vi "Create Framework.vi"(8 "error in (no error)":errorcluster, 11 "Application Data in":T1) -> (0 "error out":errorcluster, 2 "new item tag":string, 3 "Application Data Out":T1)   [LabVIEW 2017, in "DSF Core.lvlib"]
uses:
  DSF Core.lvlib
  Main VI/Application Data.ctl
  LabVIEW-Memory/Source/Classes/Pointer/Pointer.lvclass
  Classes/Framework/Framework.lvclass
  Buffer Reader/Buffer Data.ctl
  Classes/Buffer/Buffer.lvclass
  Classes/Transfer Group Status/Status.lvclass
  Typedefs/DSF Data Type.ctl
  Typedefs/DSF Engine Channel Configuration.ctl
  Typedefs/DSF Settings Info.ctl
  Typedefs/DSF Byte Order.ctl
  Typedefs/DSF Engine Framework Configuration.ctl
  Typedefs/DSF Engine Plugin Configuration.ctl
  Typedefs/DSF Timing Info.ctl
  Typedefs/DSF Engine Plugin Thread Configuration.ctl
  Typedefs/DSF Engine Transfer Group Configuration.ctl
  Typedefs/DSF Direction.ctl
  Typedefs/DSF Engine Transfer Configuration.ctl
  Typedefs/DSF Timeout Behavior.ctl
  Classes/Framework/Framework.lvclass/Framework.ctl
  Classes/Framework Status/Framework Status.lvclass/Framework Status.ctl
  ID to Tree Items/Tree Item Type.ctl
  Classes/Framework Status/Framework Status.lvclass
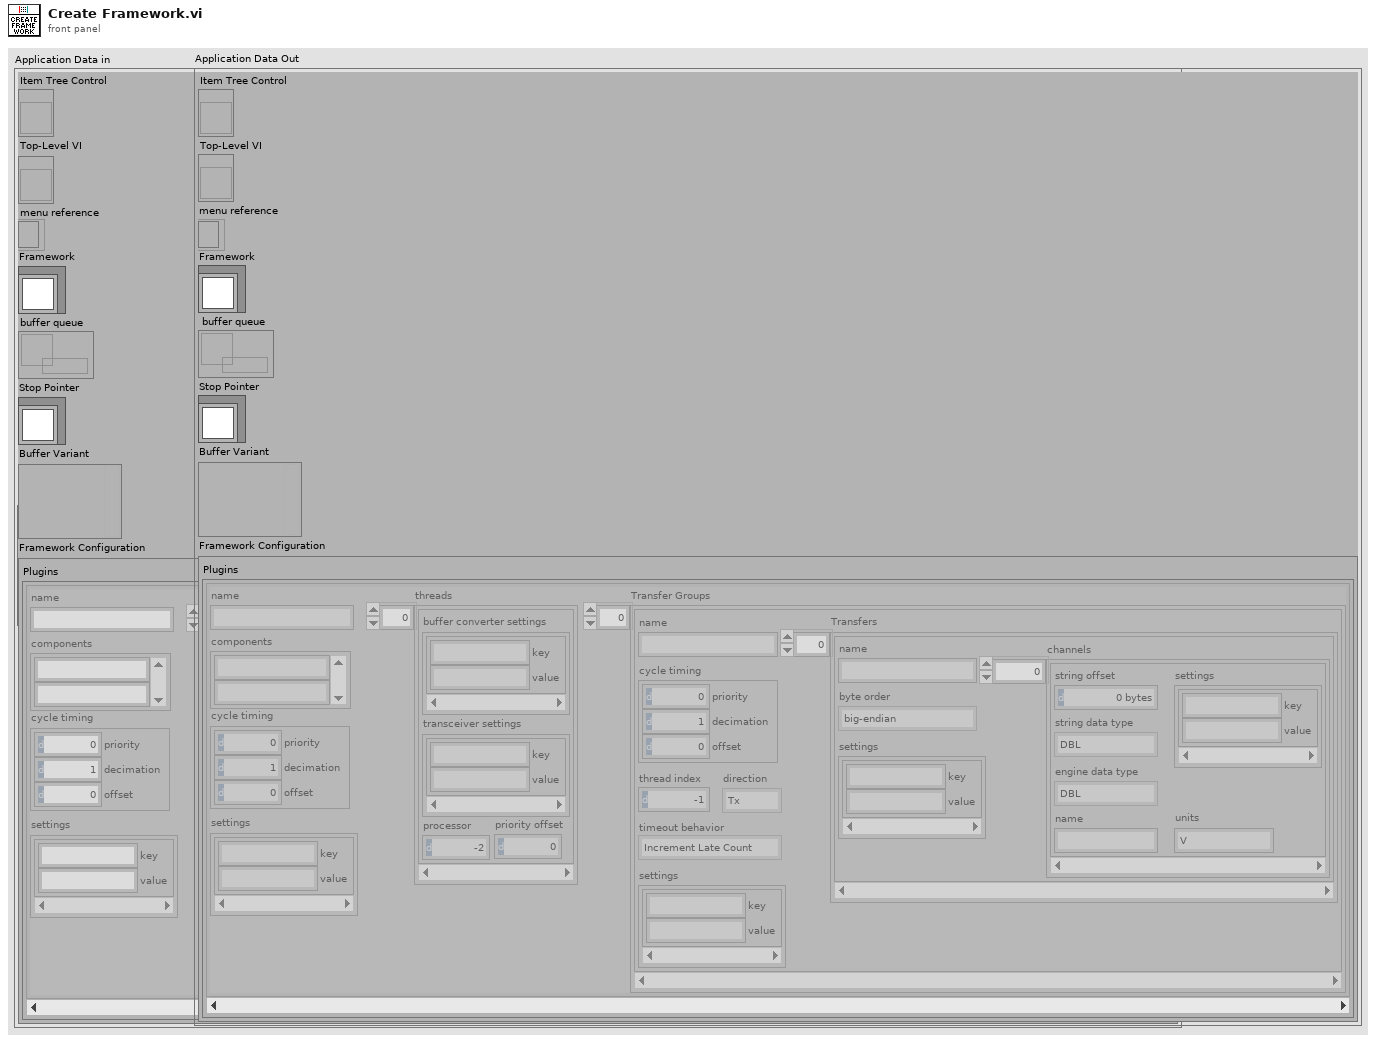
[diagram p1: front panel]
types:
  T1 = typedef "DSF Core.lvlib/Application Data.ctl" = cluster{"Item Tree Control":refnum<vi>, "Top-Level VI":refnum<vi>, "menu reference":refnum<k9>, "Framework":refnum<class "Framework.lvclass">, "buffer queue":refnum<queue>, "Stop Pointer":refnum<class "Pointer.lvclass">, "Buffer Variant":variant, "Framework Configuration":T2}
  T2 = typedef "DSF Core.lvlib/DSF Engine Framework Configuration.ctl" = cluster{"Plugins":T3[]}
  T3 = typedef "DSF Core.lvlib/DSF Engine Plugin Configuration.ctl" = cluster{"name":string, "components":string[], "cycle timing":T4, "threads":T5[], "Transfer Groups":T7[], "settings":T6}
  T4 = typedef "DSF Core.lvlib/DSF Timing Info.ctl" = cluster{"priority":u64, "decimation":u64, "offset":u64}
  T5 = typedef "DSF Core.lvlib/DSF Engine Plugin Thread Configuration.ctl" = cluster{"buffer converter settings":T6, "transceiver settings":T6, "processor":i32, "priority offset":i16}
  T6 = typedef "DSF Core.lvlib/DSF Settings Info.ctl" = cluster{"key":string, "value":string}[]
  T7 = typedef "DSF Core.lvlib/DSF Engine Transfer Group Configuration.ctl" = cluster{"name":string, "direction":T8, "cycle timing":T4, "thread index":i32, "settings":T6, "Transfers":T9[], "timeout behavior":T13}
  T8 = typedef "DSF Core.lvlib/DSF Direction.ctl" = enum8{"Tx", "Rx"}
  T9 = typedef "DSF Core.lvlib/DSF Engine Transfer Configuration.ctl" = cluster{"name":string, "byte order":T10, "settings":T6, "channels":T11[]}
  T10 = typedef "DSF Core.lvlib/DSF Byte Order.ctl" = enum8{"big-endian", "little-endian"}
  T11 = typedef "DSF Core.lvlib/DSF Engine Channel Configuration.ctl" = cluster{"string offset":u64, "string data type":T12, "engine data type":T12, "name":string, "settings":T6, "units":string}
  T12 = typedef "DSF Core.lvlib/DSF Data Type.ctl" = enum8{"Bool", "SGL", "DBL", "I8", "I16", "I32", "I64", "U8", "U16", "U32", "U64"}
  T13 = typedef "DSF Core.lvlib/DSF Timeout Behavior.ctl" = enum8{"Increment Late Count", "Throw Error"}
  T14 = typedef "DSF Core.lvlib/Buffer Data.ctl" = cluster{"Buffer":refnum<class "Buffer.lvclass">, "Status":refnum<class "Status.lvclass">, "decimation":u64, "avg bandwidth":dbl, "data type":T12, "units":string, "channels":T11[], "channel":bool, "engine (T) / string (F)":bool, "byte order":T10}
  T15 = typedef "DSF Core.lvlib/Tree Item Type.ctl" = enum16{"Framework", "Plugin Group", "Plugin", "Group", "Transfer", "Buffer", "Channel"}
  T16 = typedef "DSF Core.lvlib/Tree Item.ctl" = cluster{"Left Cell String":string, "Child Text":string[], "Child Tag":string, "Glyph Index":i32}
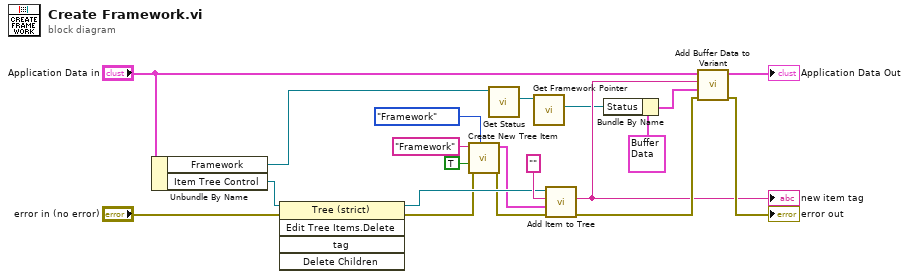
[diagram p0: block diagram]
diagram:
  n1 = Unbundle By Name("Application Data in") -> ("Framework"=w4:refnum<class "Framework.lvclass">, "Item Tree Control"=w12:refnum<vi>)
  n2 = invoke class="Tree (strict)" method="Edit Tree Items.Delete"(reference=w12, error in="error in (no error)") -> (reference out=w19:refnum<vi>, error out=w18:errorcluster)  [unwired: 3 in, 3 out]
  n3 = call "Create New Tree Item.vi"("Item Type"=Tree_Item_Type."Framework", "error in"=w18, "found?"=TRUE, "Left Cell String"="Framework") -> ("error out"=w17:errorcluster, "Item"=w16:T16)  [unwired: 6 in]
  n4 = call "Get Status.vi"("Framework in"=w4) -> ("Status"=w3:refnum<class "Framework Status.lvclass">)  [unwired: 9 in, 1 out]
  n5 = call "Get Framework Pointer.vi"("Framework Status in"=w3) -> ("framework pointer"=w2:refnum<class "Status.lvclass">)  [unwired: 9 in, 1 out]
  n6 = call "Add Item to Tree.vi"("error in (no error)"=w17, "Item"=w16, "parent tag"="", "TreeControl in"=w19) -> ("error out"=w7:errorcluster, "new item tag"=w6:string)  [unwired: 5 in, 1 out]
  "new item tag" <- w6
  n7 = Bundle By Name(cluster=T14 {"Buffer"=refnum, "Status"=refnum, "decimation"=0, "avg bandwidth"=0.0, "data type"=enum."Bool", "units"="", "channels"=[], "channel"=FALSE, "engine (T) / string (F)"=FALSE, "byte order"=enum."little-endian"} ("Buffer data"), "Status"=w2) -> (w1:T14)
  n8 = call "Add Buffer Data to Variant.vi"("error in (no error)"=w7, "Buffer data"=w1, "tag"=w6, "Application Data In in"="Application Data in") -> ("error out"=→"error out":errorcluster, "Application Data In out"=→"Application Data Out":T1)  [unwired: 6 in]
